vi "ConvertSensitivityStringtoDouble.vi"(1 "Sensitivity":string) -> (0 "Sensitivtiy":dbl)   [LabVIEW 2016, in "SR7270 Drivers.lvclass"]
uses:
  SR7270 Drivers.lvclass
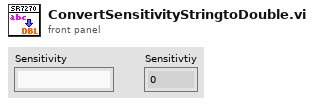
[diagram p1: front panel]
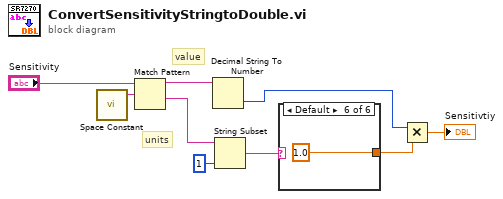
[diagram p0: block diagram]
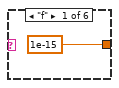
[diagram p2: hidden frame]
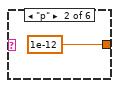
[diagram p3: hidden frame]
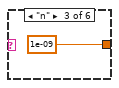
[diagram p4: hidden frame]
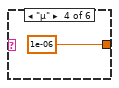
[diagram p5: hidden frame]
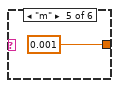
[diagram p6: hidden frame]
diagram:
  # "value"
  # "units"
  n1 = call <vilib>:"Space Constant.vi"() -> ("String"=w1:string)
  n2 = Match Pattern(string="Sensitivity", regular expression=w1) -> (before substring=w2:string, after substring=w3:string)  [unwired: 1 in, 2 out]
  n3 = Decimal String To Number(string=w2) -> (number=w7:i32)  [unwired: 2 in, 1 out]
  n4 = String Subset(string=w3, length (rest)=1 ("length (rest)")) -> (substring=w5:string)  [unwired: 1 in]
  n5 = case shown="Default" w5 {
    tunnel: [1e-15 1e-12 1e-09 1e-06 0.001 1.0] -> w6
    frame "f" {
    }
    frame "p" {
    }
    frame "n" {
    }
    frame "µ" {
    }
    frame "m" {
    }
    frame Default {
    }
  }
  n6 = Multiply(x=w7, y=w6) -> (x*y=→"Sensitivtiy":dbl)
